vi "Get DATA.vi"(8 "error in":errorcluster, 11 "axis in":cluster{"keyHandle":u32, "nodeId":u16}={"keyHandle"=262145, "nodeId"=1}) -> (0 "error out":errorcluster, 3 "axis out":cluster{"keyHandle":u32, "nodeId":u16}={"keyHandle"=262145, "nodeId"=1})   [LabVIEW 2019, in "maxonEPOS.lvlib"]
uses:
  maxonEPOS.lvlib
panel:
  in  "Boolean":bool
  in  "Tab Control":T1(tab)
  out "motor Data":T2={"motor Type"=1, "continuousCurrent"=0, "peakCurrent"=0, "polePair"=0, "thermalTimeConstant"=0} {"motor Type" items=["Phase modulated DC motor "=1, "Sinusoidal PM BL motor"=10, "Trapezoidal PM BL motor"=11]}
  out "encoder parameter":cluster{"sensorType":u16, "encoder counts":u32}={"sensorType"=1, "encoder counts"=0} {"sensorType" items=["Incremental encoder (3-channel)"=1, "Incremental encoder (2-channel)"=2, "Hall sensors"=3, "SSI absolute encoder - binary coded data"=4, "SSI absolute encoder - gray coded data"=5, "Incremenatal encoder 2 (3-channel)"=6, "Incremenatal encoder 2 (2-channel)"=7, "Absolute incremental encoder (3-channel)"=8, "Absolute incremental encoder (2-channel)"=9]}
  out "Current Control Gains":cluster{"p-Gain":u16, "i-Gain":u16}
  out "Position Control Gains":T3
  out "libraryName":string="maxon motor ag - EPOS Command Library - 32-Bit"
  out "libraryVersion":string="1.0.0.0"
  out "targetReached":i32
  # "Parameter of EPOS2/4"
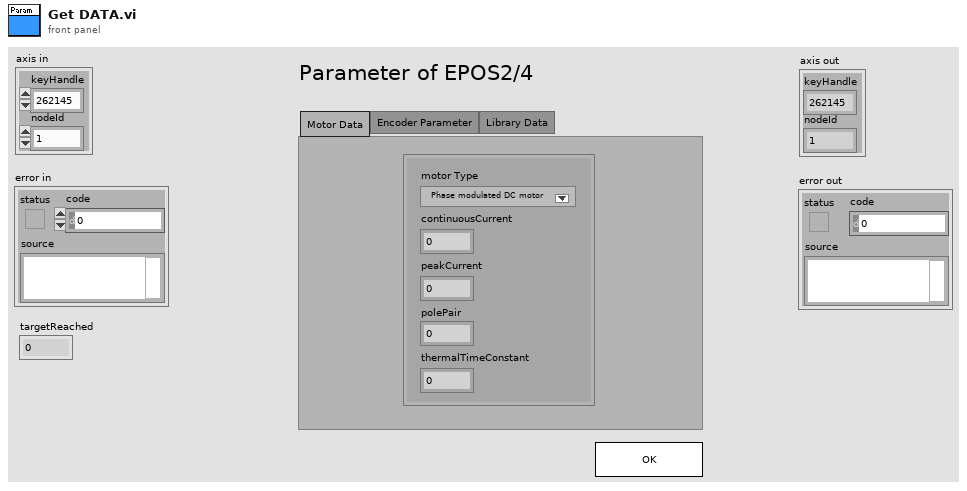
[diagram p1: front panel]
types:
  T1 = enum32{"Motor Data", "Encoder Parameter", "Control Parameter", "Library Data"}
  T2 = cluster{"motor Type":u16, "continuousCurrent":u32, "peakCurrent":u32, "polePair":u8, "thermalTimeConstant":u16}
  T3 = cluster{"p-Gain":u16, "i-Gain":u16, "d-Gain":u16}
  T4 = cluster{"nominalCurrent":u32, "maxOutputCurrent":u32, "thermalTimeConstant":u16, "nbOfPolePairs":u8}
  T5 = cluster{"motor type":u16, "nominalCurrent":u32, "maxOutputCurrent":u32, "nbOfPolePairs":u8, "thermalTimeConstant":u16}
  T6 = cluster{"nominal current":u32, "max output current":u32, "thermal time constant":u16}
  T7 = cluster{"motor type":u16, "nominal current":u32, "max output current":u32, u8, "thermal time constant":u16}
  T8 = cluster{"encoderResolution":u32, "invertedPolarity":i32}
  T9 = cluster{"sensorType":u16, "encoderResolution":u32}
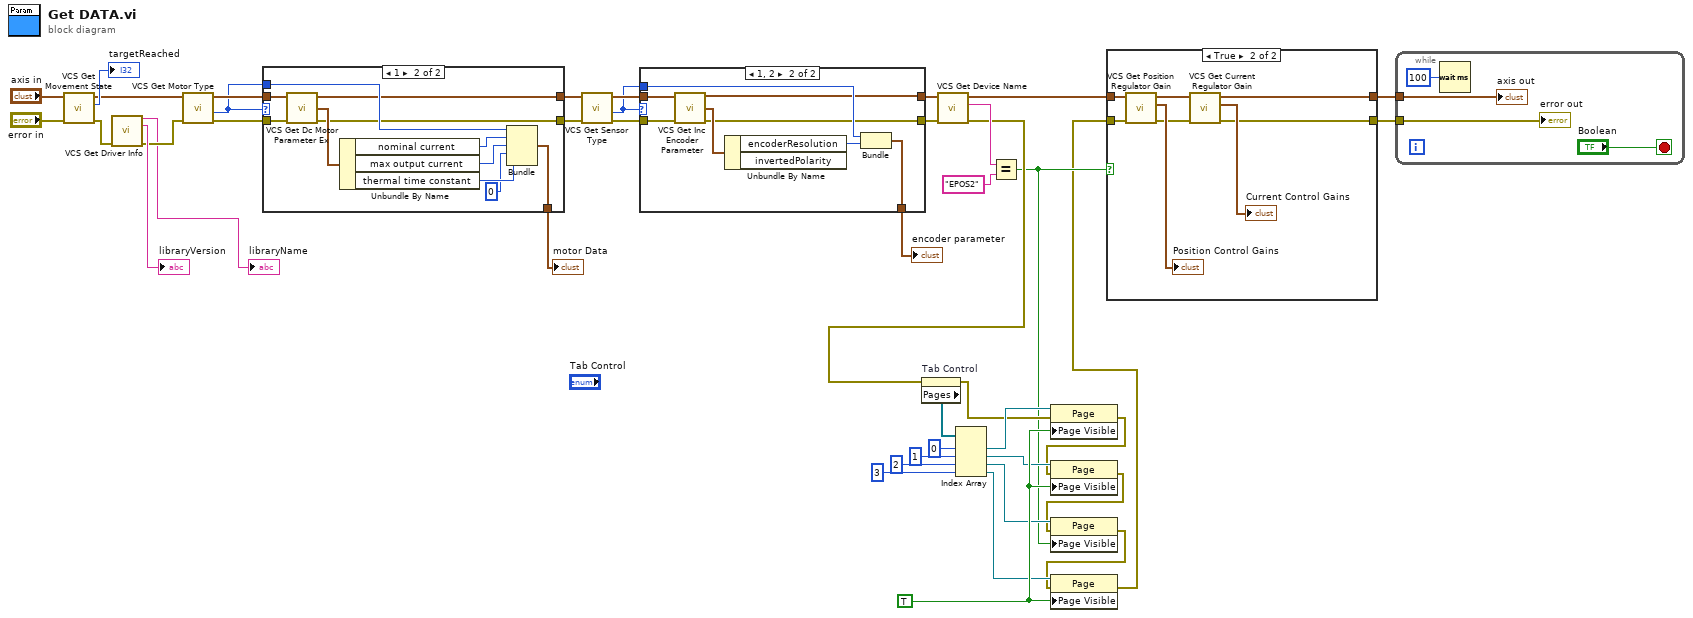
[diagram p0: block diagram]
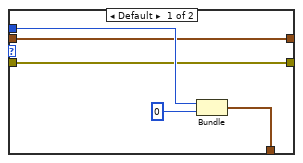
[diagram p3: hidden frame]
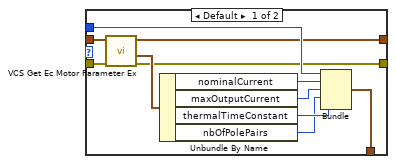
[diagram p4: hidden frame]
diagram:
  w19 = TRUE ("Page Visible")
  n1 = call "VCS Get Movement State.vi"("error in (no error)"="error in", "axis in"="axis in") -> ("error out"=w39:errorcluster, "targetReached"=→"targetReached":i32, "axis out"=w34:cluster{"keyHandle":u32, "nodeId":u16})  [unwired: 7 in]
  n2 = call "VCS Get Driver Info.vi"("error in (no error)"=w39) -> ("libraryName"=→"libraryName":string, "libraryVersion"=→"libraryVersion":string, "error out"=w35:errorcluster)  [unwired: 12 in]
  n3 = call "VCS Get Motor Type.vi"("error in (no error)"=w35, "axis in"=w34) -> ("error out"=w32:errorcluster, "motor type"=w31:u16, "axis out"=w33:cluster{"keyHandle":u32, "nodeId":u16})  [unwired: 7 in]
  n4 = case shown="1" w31 {
    tunnel: w33 -> [w47 w64]
    tunnel: w32 -> [w44 w63]
    tunnel: w31 -> [w51 w61]
    tunnel: [w50 w58] -> w30
    tunnel: [w46 w55] -> w5
    tunnel: [w43 w54] -> w4
    frame Default {
      n5 = call "VCS Get Ec Motor Parameter Ex.vi"("error in (no error)"=w44, "axis in"=w47) -> ("error out"=w43:errorcluster, "EC motor parameter ex"=w45:T4, "axis out"=w46:cluster{"keyHandle":u32, "nodeId":u16})  [unwired: 3 in]
      n6 = Unbundle By Name(w45) -> ("nominalCurrent"=w53:u32, "maxOutputCurrent"=w52:u32, "thermalTimeConstant"=w49:u16, "nbOfPolePairs"=w48:u8)
      n7 = Bundle("motor type"=w51, "nominalCurrent"=w53, "maxOutputCurrent"=w52, "nbOfPolePairs"=w48, "thermalTimeConstant"=w49) -> (w50:T5)  [unwired: 1 in]
    }
    frame 1 {
      n8 = call "VCS Get Dc Motor Parameter Ex.vi"("axis in"=w64, "error in (no error)"=w63) -> ("axis out"=w55:cluster{"keyHandle":u32, "nodeId":u16}, "DC motor parameter ex"=w62:T6, "error out"=w54:errorcluster)  [unwired: 11 in]
      n9 = Unbundle By Name(w62) -> ("nominal current"=w60:u32, "max output current"=w59:u32, "thermal time constant"=w57:u16)
      n10 = Bundle("motor type"=w61, "nominal current"=w60, "max output current"=w59, u8 0, "thermal time constant"=w57) -> (w58:T7)  [unwired: 1 in]
    }
  }
  "motor Data" <- w30
  n11 = call "VCS Get Sensor Type.vi"("error in (no error)"=w4, "axis in"=w5) -> ("error out"=w3:errorcluster, "sensorType"=w2:u16, "axis out"=w6:cluster{"keyHandle":u32, "nodeId":u16})  [unwired: 7 in]
  n12 = case shown="1, 2" w2 {
    tunnel: w3 -> [w65 w77]
    tunnel: w6 -> [w66 w76]
    tunnel: w2 -> [w68 w74]
    tunnel: [w69 w73] -> w1
    tunnel: [w66 w71] -> w26
    tunnel: [w65 w70] -> w28
    frame Default {
      n13 = Bundle("sensorType"=w68, u32 0) -> (w69:cluster{"sensorType":u16, u32})  [unwired: 1 in]
    }
    frame 1, 2 {
      n14 = call "VCS Get Inc Encoder Parameter.vi"("axis in"=w76, "error in (no error)"=w77) -> ("axis out"=w71:cluster{"keyHandle":u32, "nodeId":u16}, "incremental encoder parameter"=w75:T8, "error out"=w70:errorcluster)  [unwired: 11 in]
      n15 = Unbundle By Name(w75) -> ("encoderResolution"=w72:u32)  [unwired: 1 out]
      n16 = Bundle("sensorType"=w74, "encoderResolution"=w72) -> (w73:T9)  [unwired: 1 in]
    }
  }
  "encoder parameter" <- w1
  n17 = call "VCS Get Device Name.vi"("error in (no error)"=w28, "axis in"=w26) -> ("error out"=w9:errorcluster, "deviceName"=w24:string, "axis out"=w27:cluster{"keyHandle":u32, "nodeId":u16})  [unwired: 7 in]
  n18 = property on="Tab Control" class="TabCtl (strict)"(error in=w9) -> (error out=w13:errorcluster, "Pages"=w17:refnum<vi>[])  [unwired: 1 in, 1 out]
  n19 = Index Array(array=w17, index #1=0 ("index"), index #2=1 ("index"), index #3=2 ("index"), index #4=3 ("index")) -> (element #1=w18:refnum<vi>, element #2=w16:refnum<vi>, element #3=w15:refnum<vi>, element #4=w14:refnum<vi>)
  n20 = Equal?(x=w24, y="EPOS2" ("x")) -> (x = y?=w8:bool)
  n21 = property class="Page"(reference=w18, error in=w13, "Page Visible"=w19) -> (error out=w12:errorcluster)  [unwired: 1 out]
  n22 = property class="Page"(reference=w16, error in=w12, "Page Visible"=w19) -> (error out=w11:errorcluster)  [unwired: 1 out]
  n23 = property class="Page"(reference=w15, error in=w11, "Page Visible"=w8) -> (error out=w10:errorcluster)  [unwired: 1 out]
  n24 = property class="Page"(reference=w14, error in=w10, "Page Visible"=w19) -> (error out=w7:errorcluster)  [unwired: 1 out]
  n25 = case shown="True" w8 {
    tunnel: [w79 w83] -> w37
    tunnel: [w78 w82] -> w36
    tunnel: w7 -> [w78 w81]
    tunnel: w27 -> [w79 w80]
    frame False {
    }
    frame True {
      n26 = call "VCS Get Position Regulator Gain.vi"("error in (no error)"=w81, "axis in"=w80) -> ("error out"=w84:errorcluster, "gains"=→"Position Control Gains":T3, "axis out"=w85:cluster{"keyHandle":u32, "nodeId":u16})  [unwired: 7 in]
      n27 = call "VCS Get Current Regulator Gain.vi"("error in (no error)"=w84, "axis in"=w85) -> ("error out"=w82:errorcluster, "gains"=→"Current Control Gains":cluster{"p-Gain":u16, "i-Gain":u16}, "axis out"=w83:cluster{"keyHandle":u32, "nodeId":u16})  [unwired: 7 in]
    }
  }
  n28 = while {
    tunnel: w37 -> [w91]
    tunnel: w36 -> [w90]
    stop <- "Boolean" stop-if-true
    n29 = Wait (ms)(milliseconds to wait=u32 100) -> ()  [unwired: 1 out]
    "error out" <- w90
    "axis out" <- w91
  }
